vi "CloseNode.vi"(8 "error in":errorcluster, 11 "node ref":T1) -> (0 "error out":errorcluster)   [LabVIEW 2013, in "NISE_CEF_TreeControl.lvlib"]
doc: "This is the node Clean Up Vi it will close all the open references for the node and its childs"
uses:
  NISE_CEF_TreeControl.lvlib
  Node/NodeRef.ctl
  Node/NISE_CEF_Node.lvclass
  Node/NISE_CEF_Node.lvclass/NISE_CEF_Node.ctl
  Node/ReadChildren.vi
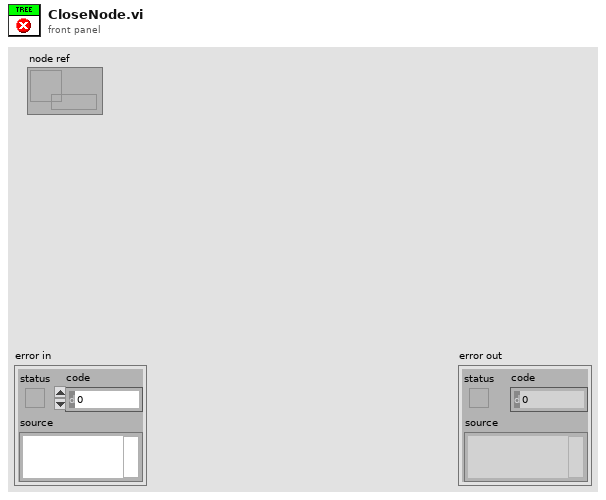
[diagram p1: front panel]
types:
  T1 = typedef "NISE_CEF_Node.lvclass/NodeRef.ctl" = refnum<data-value>
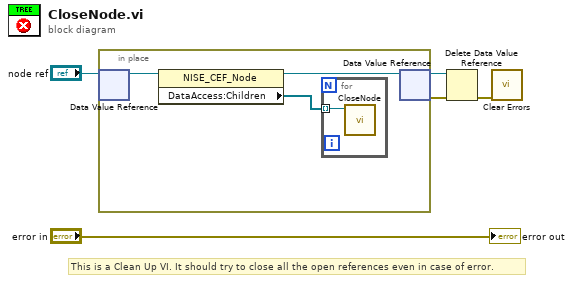
[diagram p0: block diagram]
diagram:
  # "This is a Clean Up VI. It should try to close all the open references even in case of error."
  n1 = in-place {
    n2 = in-place-dvr #1("node ref") -> (w8:refnum<class "NISE_CEF_Node.lvclass">)  [unwired: 1 out]
    n3 = property class="NISE_CEF_Node"(reference=w8) -> (reference out=w6:refnum<class "NISE_CEF_Node.lvclass">, "DataAccess:Children"=w7:T1[])  [unwired: 1 in, 1 out]
    n4 = for {
      tunnel: w7 -> [w9] mode=indexing
      n5 = call "CloseNode.vi"("node ref"=w9) -> ()  [unwired: 10 in, 1 out]
    }
    n6 = in-place-dvr #1(w6) -> (w4:T1, w2:errorcluster)
  }
  n7 = Delete Data Value Reference(data value reference=w4, error in=w2) -> (error out=w1:errorcluster)  [unwired: 1 out]
  n8 = call <vilib>:"Clear Errors.vi"("error in (no error)"=w1) -> ()  [unwired: 6 in, 1 out]
  "error out" <- "error in"
